vi "NT Read String.vi"(8 "error in":errorcluster, 9 "Default Value":string, 11 "Name":string="String") -> (0 "error out":errorcluster, 3 "String":string)   [LabVIEW 2017]
doc: "Return the string stored in the named entry. Return an error if not present or not a string. Names that begin with a slash character \"/\" specify a full path, otherwise they are relative to /SmartDashboard/."
uses:
  <vilib>/Rock Robotics/Network Tables/Field Type.ctl
  <vilib>/Rock Robotics/Network Tables/Create Actual Table Name.vi
  <vilib>/Rock Robotics/Network Tables/Field Data Manager.vi
  <vilib>/Rock Robotics/Network Tables/Table Manager.vi
  <vilib>/Rock Robotics/Network Tables/Usage Statistics.vi
  <vilib>/Rock Robotics/Network Tables/NT Globals.vi
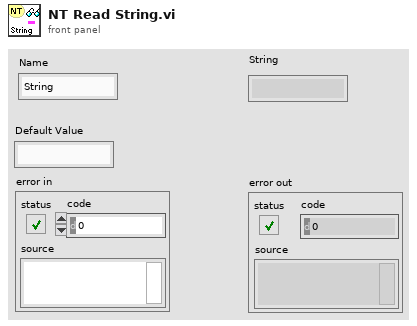
[diagram p1: front panel]
types:
  T1 = typedef "Field Type.ctl" = enum8{"Invalid", "Bool", "Numeric", "String", "Raw", "Boolean Array", "Numeric Array", "String Array", "RPC"}
  T2 = typedef "Field Data.ctl" = cluster{"Dbl":dbl, "String":string, "Type":T1, "Boolean":bool, "Sequence #":T3, "Flags":u8}
  T3 = typedef "Sequence.ctl" = u16
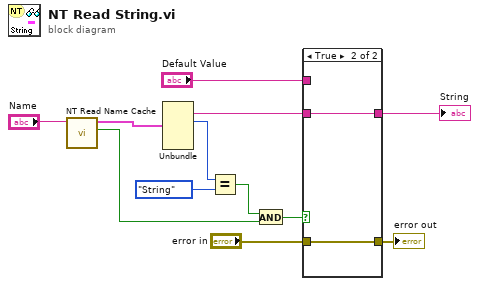
[diagram p0: block diagram]
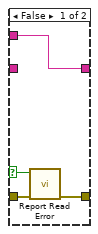
[diagram p2: hidden frame]
diagram:
  n1 = call <vilib>:"NT Read Name Cache.vi"("Name"="Name") -> ("Success"=w6:bool, "Field Value Out"=w7:T2)  [unwired: 9 in]
  n2 = Unbundle(w7) -> ("String"=w2:string, "Type"=w10:T1)  [unwired: 4 out]
  n3 = Equal?(x=w10, y=Field_Type."String" ("Type")) -> (x = y?=w12:bool)
  n4 = And(x=w12, y=w6) -> (x .and. y?=w4:bool)
  n5 = case shown="True" w4 {
    selector: w4 -> [w14 _]
    tunnel: [w16 w18] -> w9
    tunnel: "error in" -> [w15 w18]
    tunnel: "Default Value" -> [w13 _]
    tunnel: w2 -> [_ w17]
    tunnel: [w13 w17] -> w1
    frame False {
      n6 = call <vilib>:"Report Read Error.vi"("error in (no error)"=w15, "Success"=w14) -> ("error out"=w16:errorcluster)  [unwired: 9 in]
    }
    frame True {
    }
  }
  "String" <- w1
  "error out" <- w9
